vi "poly test (double).vi"(1 "x":dbl) -> (0 "x+1":dbl)   [LabVIEW 2013]
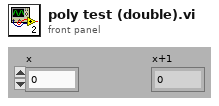
[diagram p1: front panel]
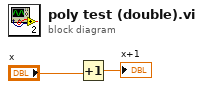
[diagram p0: block diagram]
diagram:
  n1 = Increment(x="x") -> (x+1=→"x+1":dbl)
